vi "CarWash-Simulator.vi"   [LabVIEW 2021]
uses:
  Global-Var-Simulator.vi
  Global-Var-ControlPanel.vi
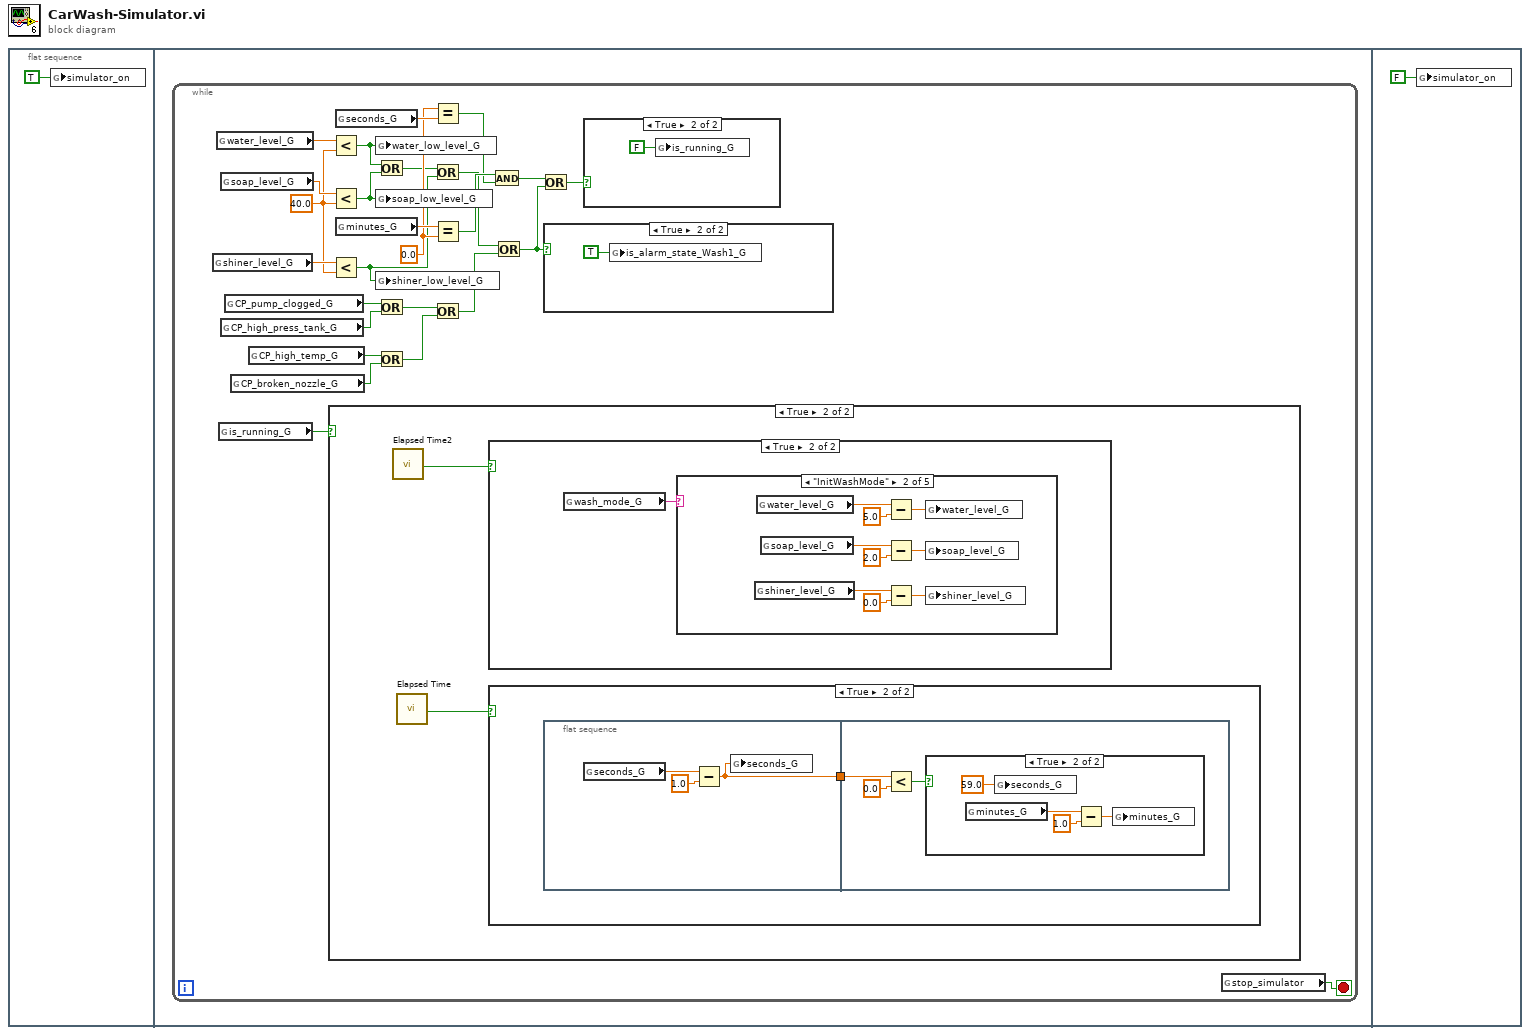
[diagram p0: block diagram]
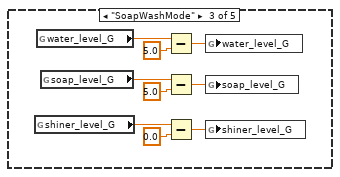
[diagram p7: hidden frame]
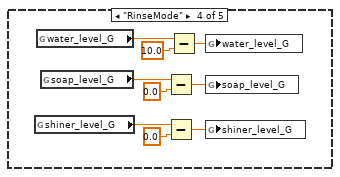
[diagram p8: hidden frame]
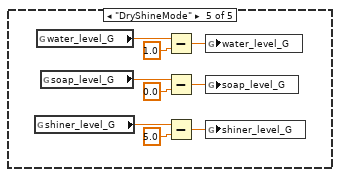
[diagram p9: hidden frame]
diagram:
  n1 = flat-sequence {
    frame #0 {
      n2 = global write "Global-Var-Simulator.vi" "simulator_on"(TRUE ("simulator_on")) -> ()
    }
    frame #1 {
      n3 = while {
        stop <- w18 stop-if-true
        w14 = 40.0 ("y")
        w24 = 0.0 ("y")
        n4 = global read "Global-Var-Simulator.vi" "shiner_level_G"() -> (w15:dbl)
        n5 = global read "Global-Var-Simulator.vi" "water_level_G"() -> (w17:dbl)
        n6 = global read "Global-Var-Simulator.vi" "is_running_G"() -> (w27:bool)
        n7 = global read "Global-Var-Simulator.vi" "soap_level_G"() -> (w16:dbl)
        n8 = global read "Global-Var-ControlPanel.vi" "CP_high_press_tank_G"() -> (w7:bool)
        n9 = global read "Global-Var-ControlPanel.vi" "CP_pump_clogged_G"() -> (w8:bool)
        n10 = global read "Global-Var-ControlPanel.vi" "CP_broken_nozzle_G"() -> (w9:bool)
        n11 = global read "Global-Var-ControlPanel.vi" "CP_high_temp_G"() -> (w10:bool)
        n12 = case shown="True" w27 {
          frame False {
          }
          frame True {
            n13 = call "Elapsed Time2"() -> ("Time has Elapsed"=w30:bool)  [unwired: 12 in, 7 out]
            n14 = call "Elapsed Time"() -> ("Time has Elapsed"=w31:bool)  [unwired: 12 in, 7 out]
            n15 = case shown="True" w30 {
              frame False {
              }
              frame True {
                n16 = global read "Global-Var-Simulator.vi" "wash_mode_G"() -> (w32:string)
                n17 = case shown="\"InitWashMode\"" w32 {
                  frame "NoneWashMode", Default {
                  }
                  frame "InitWashMode" {
                    n18 = global read "Global-Var-Simulator.vi" "shiner_level_G"() -> (w35:dbl)
                    n19 = global read "Global-Var-Simulator.vi" "water_level_G"() -> (w41:dbl)
                    n20 = global read "Global-Var-Simulator.vi" "soap_level_G"() -> (w38:dbl)
                    n21 = Subtract(x=w41, y=5.0) -> (x-y=w39:dbl)
                    n22 = Subtract(x=w38, y=2.0) -> (x-y=w36:dbl)
                    n23 = Subtract(x=w35, y=0.0) -> (x-y=w34:dbl)
                    n24 = global write "Global-Var-Simulator.vi" "water_level_G"(w39) -> ()
                    n25 = global write "Global-Var-Simulator.vi" "soap_level_G"(w36) -> ()
                    n26 = global write "Global-Var-Simulator.vi" "shiner_level_G"(w34) -> ()
                  }
                  frame "SoapWashMode" {
                    n27 = global read "Global-Var-Simulator.vi" "shiner_level_G"() -> (w44:dbl)
                    n28 = global read "Global-Var-Simulator.vi" "water_level_G"() -> (w50:dbl)
                    n29 = global read "Global-Var-Simulator.vi" "soap_level_G"() -> (w47:dbl)
                    n30 = Subtract(x=w50, y=5.0) -> (x-y=w48:dbl)
                    n31 = Subtract(x=w47, y=5.0) -> (x-y=w45:dbl)
                    n32 = Subtract(x=w44, y=0.0) -> (x-y=w43:dbl)
                    n33 = global write "Global-Var-Simulator.vi" "water_level_G"(w48) -> ()
                    n34 = global write "Global-Var-Simulator.vi" "soap_level_G"(w45) -> ()
                    n35 = global write "Global-Var-Simulator.vi" "shiner_level_G"(w43) -> ()
                  }
                  frame "RinseMode" {
                    n36 = global read "Global-Var-Simulator.vi" "shiner_level_G"() -> (w53:dbl)
                    n37 = global read "Global-Var-Simulator.vi" "water_level_G"() -> (w59:dbl)
                    n38 = global read "Global-Var-Simulator.vi" "soap_level_G"() -> (w56:dbl)
                    n39 = Subtract(x=w56, y=0.0) -> (x-y=w54:dbl)
                    n40 = Subtract(x=w53, y=0.0) -> (x-y=w52:dbl)
                    n41 = Subtract(x=w59, y=10.0) -> (x-y=w57:dbl)
                    n42 = global write "Global-Var-Simulator.vi" "water_level_G"(w57) -> ()
                    n43 = global write "Global-Var-Simulator.vi" "soap_level_G"(w54) -> ()
                    n44 = global write "Global-Var-Simulator.vi" "shiner_level_G"(w52) -> ()
                  }
                  frame "DryShineMode" {
                    n45 = global read "Global-Var-Simulator.vi" "shiner_level_G"() -> (w62:dbl)
                    n46 = global read "Global-Var-Simulator.vi" "water_level_G"() -> (w68:dbl)
                    n47 = global read "Global-Var-Simulator.vi" "soap_level_G"() -> (w65:dbl)
                    n48 = Subtract(x=w68, y=1.0) -> (x-y=w66:dbl)
                    n49 = Subtract(x=w65, y=0.0) -> (x-y=w63:dbl)
                    n50 = Subtract(x=w62, y=5.0) -> (x-y=w61:dbl)
                    n51 = global write "Global-Var-Simulator.vi" "water_level_G"(w66) -> ()
                    n52 = global write "Global-Var-Simulator.vi" "soap_level_G"(w63) -> ()
                    n53 = global write "Global-Var-Simulator.vi" "shiner_level_G"(w61) -> ()
                  }
                }
              }
            }
            n54 = case shown="True" w31 {
              frame False {
              }
              frame True {
                n55 = flat-sequence {
                  tunnel: [w70] -> w69
                  tunnel: w69 -> [w75]
                  frame #0 {
                    n56 = global read "Global-Var-Simulator.vi" "seconds_G"() -> (w71:dbl)
                    n57 = Subtract(x=w71, y=1.0) -> (x-y=w70:dbl)
                    n58 = global write "Global-Var-Simulator.vi" "seconds_G"(w70) -> ()
                  }
                  frame #1 {
                    n59 = Less?(x=w75, y=0.0) -> (x < y?=w73:bool)
                    n60 = case shown="True" w73 {
                      frame False {
                      }
                      frame True {
                        n61 = global read "Global-Var-Simulator.vi" "minutes_G"() -> (w78:dbl)
                        n62 = global write "Global-Var-Simulator.vi" "seconds_G"(59.0 ("seconds_G")) -> ()
                        n63 = Subtract(x=w78, y=1.0) -> (x-y=w76:dbl)
                        n64 = global write "Global-Var-Simulator.vi" "minutes_G"(w76) -> ()
                      }
                    }
                  }
                }
              }
            }
          }
        }
        n65 = Less?(x=w17, y=w14) -> (x < y?=w13:bool)
        n66 = Less?(x=w16, y=w14) -> (x < y?=w12:bool)
        n67 = Less?(x=w15, y=w14) -> (x < y?=w11:bool)
        n68 = global read "Global-Var-Simulator.vi" "seconds_G"() -> (w26:dbl)
        n69 = global read "Global-Var-Simulator.vi" "minutes_G"() -> (w25:dbl)
        n70 = global write "Global-Var-Simulator.vi" "water_low_level_G"(w13) -> ()
        n71 = global write "Global-Var-Simulator.vi" "soap_low_level_G"(w12) -> ()
        n72 = global write "Global-Var-Simulator.vi" "shiner_low_level_G"(w11) -> ()
        n73 = Or(x=w13, y=w12) -> (x .or. y?=w21:bool)
        n74 = Or(x=w8, y=w7) -> (x .or. y?=w5:bool)
        n75 = Or(x=w10, y=w9) -> (x .or. y?=w6:bool)
        n76 = Equal?(x=w24, y=w26) -> (x = y?=w22:bool)
        n77 = Or(x=w21, y=w11) -> (x .or. y?=w4:bool)
        n78 = Equal?(x=w25, y=w24) -> (x = y?=w23:bool)
        n79 = Or(x=w5, y=w6) -> (x .or. y?=w3:bool)
        n80 = And(x=w23, y=w22) -> (x .and. y?=w20:bool)
        n81 = Or(x=w4, y=w3) -> (x .or. y?=w2:bool)
        n82 = Or(x=w20, y=w2) -> (x .or. y?=w19:bool)
        n83 = case shown="True" w2 {
          frame False {
          }
          frame True {
            n84 = global write "Global-Var-Simulator.vi" "is_alarm_state_Wash1_G"(TRUE ("is_running_G")) -> ()
          }
        }
        n85 = case shown="True" w19 {
          frame False {
          }
          frame True {
            n86 = global write "Global-Var-Simulator.vi" "is_running_G"(FALSE ("is_running_G")) -> ()
          }
        }
        n87 = global read "Global-Var-Simulator.vi" "stop_simulator"() -> (w18:bool)
      }
    }
    frame #2 {
      n88 = global write "Global-Var-Simulator.vi" "simulator_on"(FALSE ("simulator_on")) -> ()
    }
  }
